vi "_String with ASCII code conversion.vi"(0 "Input string":string) -> (14 "Output string":string)   [LabVIEW 2014]
doc: "Converts each ASCII control code from Input string\nto \"\\x\" with x being the ASCII code of the corresponding\ncharacter for better readability of log files. \n\nValid for: all systems"
panel:
  # "Converts each ASCII control code from Input string\nto \"\\x\" with x being the ASCII code of the corresponding\ncharacter for better readability of log files."
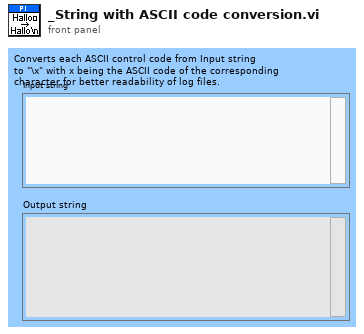
[diagram p1: front panel]
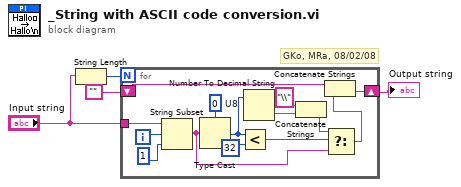
[diagram p0: block diagram]
diagram:
  # "GKo, MRa, 08/02/08"
  n1 = String Length(string="Input string") -> (length=w1:i32)
  n2 = for {
    N: w1 -> [_]
    tunnel: "Input string" -> [w18]
    shift-right: [w5] -> w4
    shift-left: "" -> [w6]
    i -> [w17]
    w15 = u8 0  # U8
    n3 = String Subset(string=w18, offset (0)=w17, length (rest)=1 ("length (rest)")) -> (substring=w12:string)
    n4 = Type Cast(type=w15, x=w12) -> (*(type *) &x=w11:u8)
    n5 = Less?(x=w11, y=u8 32 ("upper limit")) -> (x < y?=w13:bool)
    n6 = Number To Decimal String(number=w11) -> (decimal integer string=w10:string)  [unwired: 1 in]
    n7 = Concatenate Strings("\\" ("string"), w10) -> (w8:string)
    n8 = Select(t=w8, s=w13, f=w12) -> (s? t:f=w7:string)
    n9 = Concatenate Strings(w6, w7) -> (w5:string)
  }
  "Output string" <- w4
